vi "Combined Algorithm.vi"() -> ()   [LabVIEW 2020]
uses:
  <vilib>/MakerHub/LINX/Private/Type Defs/Peripherals/SPI/SPI Configuration.ctl
  <vilib>/MakerHub/LINX/Private/Type Defs/Peripherals/SPI/SPI Bit Order.ctl
  <vilib>/MakerHub/LINX/Private/Type Defs/Peripherals/SPI/SPI Mode.ctl
  <vilib>/MakerHub/LINX/Public/Peripherals/SPI/SPI CS Config.ctl
  <vilib>/MakerHub/LINX/Private/Type Defs/Peripherals/SPI/SPI CS Logic Level.ctl
  <vilib>/MakerHub/LINX/Public/Peripherals/Analog/Analog Read 1 Chan.vi
  <vilib>/MakerHub/LINX/Public/Peripherals/Digital/Digital Write 1 Chan.vi
  <vilib>/MakerHub/LINX/Public/Peripherals/SPI/SPI Write Read 1 Frame.vi
  <vilib>/MakerHub/LINX/Public/Peripherals/PWM/PWM Set Duty Cycle 1 Chan.vi
  <vilib>/MakerHub/LINX/Public/Peripherals/Analog/Analog Read N Chans.vi
  <vilib>/MakerHub/LINX/Public/Peripherals/Digital/Digital Write N Chans.vi
  <vilib>/MakerHub/LINX/Public/Peripherals/SPI/SPI Write Read N Frames.vi
  <vilib>/MakerHub/LINX/Private/Local IO/LinxAnalogRead.vi
  <vilib>/MakerHub/LINX/Public/Utilities/Check Channel.vi
  <vilib>/MakerHub/LINX/Private/Local IO/LinxDigitalWrite.vi
  <vilib>/MakerHub/LINX/Private/Local IO/LinxSpiWriteRead.vi
  <vilib>/MakerHub/LINX/Public/Utilities/Open Serial.vi
  <vilib>/MakerHub/LINX/Private/Utilties/Generate Error.vi
  <vilib>/MakerHub/LINX/Public/Peripherals/PWM/PWM Set Duty Cycle N Chans.vi
  <vilib>/MakerHub/LINX/LMH-LINX.lvlib
panel:
  in  "Esp32 SMS Send":u8
  out "LCD Response":u8[](array[numeric])
  in  "IR Sensor Analog Channel 2":u8
  in  "DO Channel -  Exhaust Fan":u8
  in  "DO Channel - Solar Water Motor":u8
  in  "IR sensor Analog Channel (A0)":u8
  out "IR Sensor (Fire detected)":bool
  out "IR Sensor output voltage":dbl
  in  "PWM Channel - Buzzer":u8
  in  "Smoke Threshold":dbl
  out "Smoke sensor output Voltage":dbl
  in  "Smoke sensor Analog Channel(A2)":u8
  out "Temperature":dbl
  in  "stop":bool
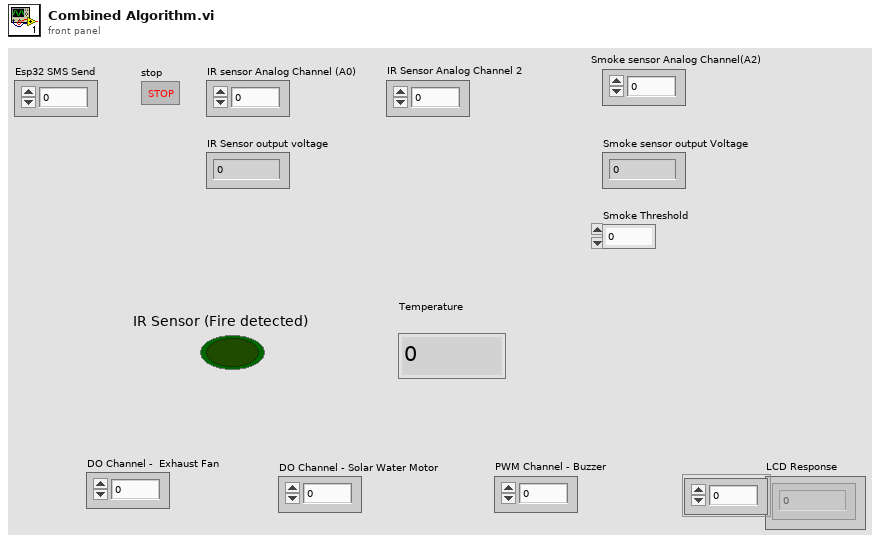
[diagram p1: front panel]
types:
  T1 = typedef "LMH-LINX.lvlib/SPI Configuration.ctl" = cluster{"Clock Frequency":u32, "Bit Order":T2, "SPI Mode":T3}
  T2 = typedef "LMH-LINX.lvlib/SPI Bit Order.ctl" = enum8{"LSb First", "MSb First"}
  T3 = typedef "LMH-LINX.lvlib/SPI Mode.ctl" = enum8{"Mode 0", "Mode 1", "Mode 2", "Mode 3"}
  T4 = typedef "LMH-LINX.lvlib/LINX Ref.ctl" = cluster{"IO":T5, "Interface":T6, "LINX Device Config":T7}
  T5 = typedef "LMH-LINX.lvlib/Platform.ctl" = enum16{"Remote", "Local"}
  T6 = typedef "LMH-LINX.lvlib/Interface.ctl" = enum16{"Serial", "TCP"}
  T7 = typedef "LMH-LINX.lvlib/Device.lvlib/LINX Device Config.ctl" = cluster{"Interface":T6, "COM Port":refnum<visa-resource-name>, "TCP Configuration":T8, "Device Family":u8, "Device ID":u8, "Device Name":string, "TCP Ref":refnum<k5>, "Channels":T9}
  T8 = typedef "LMH-LINX.lvlib/Device.lvlib/TCP Config.ctl" = cluster{"IP Address":string, "Port":u16}
  T9 = typedef "LMH-LINX.lvlib/Channels.ctl" = cluster{"DI":u8[], "DO":u8[], "AI":u8[], "AO":u8[], "PWM":u8[], "QE":u8[], "UART":u8[], "I2C 2":u8[], "SPI":u8[], "CAN":u8[], "Servo":u8[], "AI Ref (V)":dbl, "AI Resolution (Bits)":u8, "AO Ref (V)":dbl, "AO Resolution (Bits)":u8}
  T10 = typedef "LMH-LINX.lvlib/SPI CS Config.ctl" = cluster{"CS Channel":u8, "CS Logic Level":T11}
  T11 = typedef "LMH-LINX.lvlib/SPI CS Logic Level.ctl" = enum8{"Active Low", "Active High"}
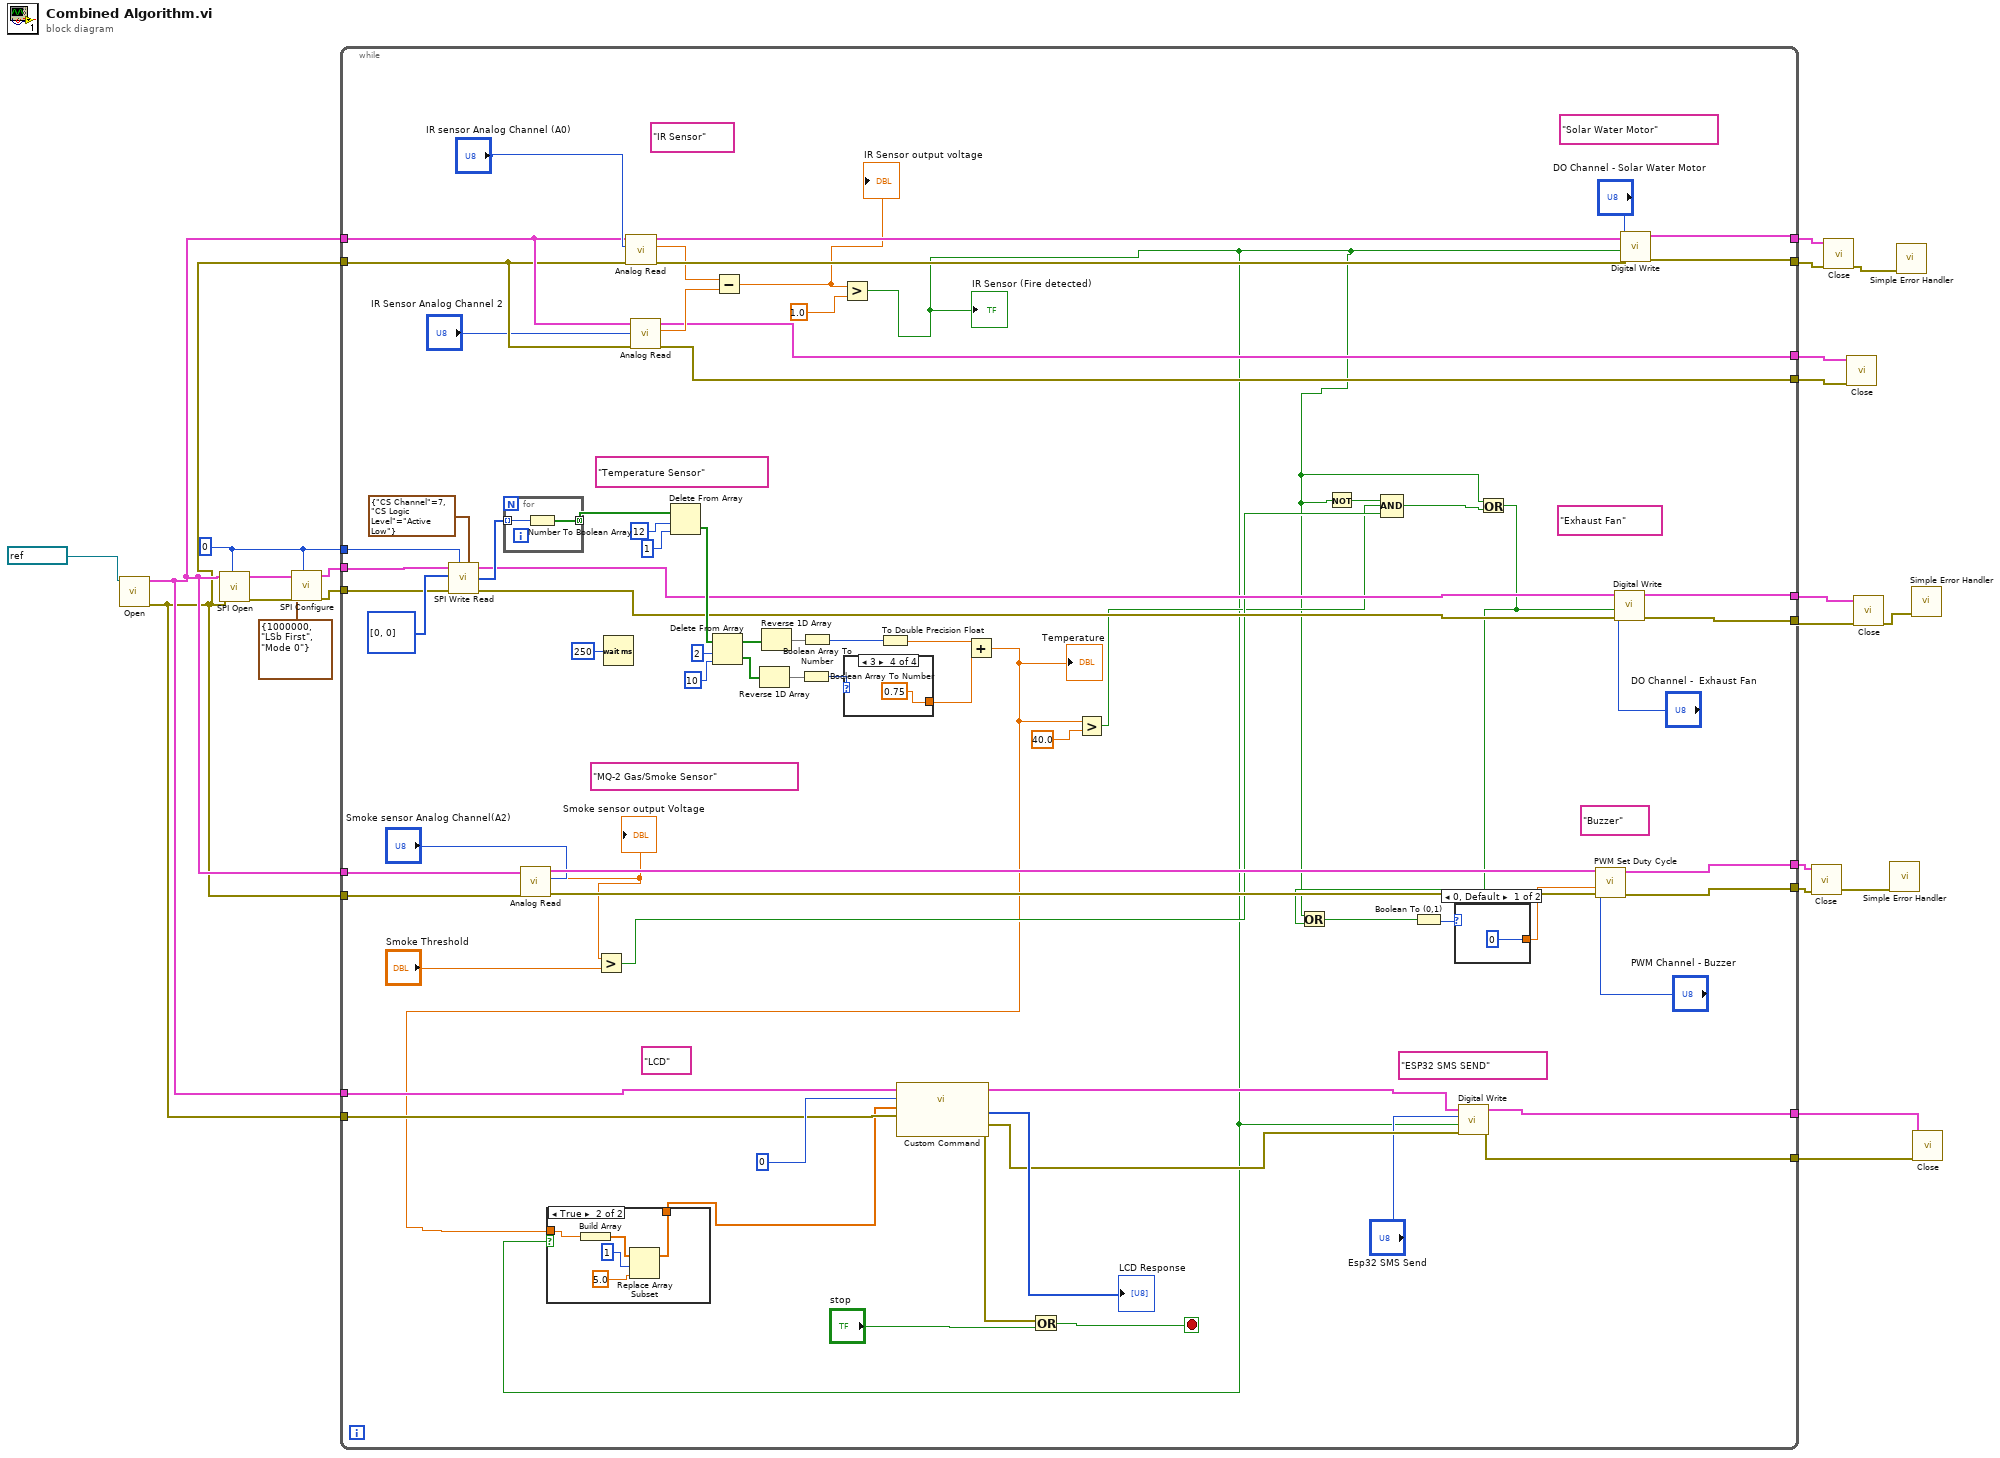
[diagram p0: block diagram]
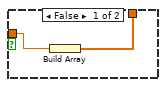
[diagram p2: hidden frame]
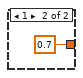
[diagram p3: hidden frame]
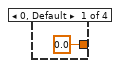
[diagram p4: hidden frame]
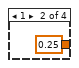
[diagram p5: hidden frame]
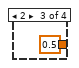
[diagram p6: hidden frame]
diagram:
  w16 = u8 0 ("SPI Channel (0)")
  n1 = call-poly <vilib>:"Open.vi"("Serial Port"=refnum<visa-resource-name> "COM3") -> ("Error Out"=w3:errorcluster, "LINX Resource"=w4:T4)  [unwired: 8 in, 1 out]
  n2 = call <vilib>:"SPI Open.vi"("SPI Channel (0)"=w16, "Error In"=w3, "LINX Resource"=w4) -> ("Error Out"=w21:errorcluster, "LINX Resource"=w20:T4)  [unwired: 7 in]
  n3 = call <vilib>:"SPI Configure.vi"("SPI Channel (0)"=w16, "Error In"=w21, "SPI Configuration"=T1 {"Clock Frequency"=1000000, "Bit Order"=enum."LSb First", "SPI Mode"=enum."Mode 0"}, "LINX Resource"=w20) -> ("Error Out"=w18:errorcluster, "LINX Resource"=w19:T4)  [unwired: 5 in, 1 out]
  n4 = while {
    tunnel: w19 -> [w95]
    tunnel: [w56] -> w10
    tunnel: w18 -> [w78]
    tunnel: [w55] -> w17
    tunnel: w16 -> [w77]
    tunnel: w4 -> [w69]
    tunnel: w3 -> [w68]
    tunnel: [w66] -> w14
    tunnel: [w65] -> w13
    tunnel: w4 -> [w46]
    tunnel: w3 -> [w45]
    tunnel: [w61] -> w12
    tunnel: [w60] -> w11
    tunnel: [w40] -> w6
    tunnel: [w39] -> w5
    tunnel: w4 -> [w34]
    tunnel: w3 -> [w33]
    tunnel: [w27] -> w2
    tunnel: [w29] -> w1
    stop <- w32 stop-if-true
    (unwired) "ESP32 SMS SEND"
    (unwired) "LCD"
    (unwired) "Exhaust Fan"
    (unwired) "Buzzer"
    (unwired) "Solar Water Motor"
    (unwired) "IR Sensor"
    (unwired) "Temperature Sensor"
    (unwired) "MQ-2 Gas/Smoke Sensor"
    n5 = call-poly <vilib>:"SPI Write Read.vi"("CS Configuration"=T10 {"CS Channel"=7, "CS Logic Level"=enum."Active Low"}, "SPI Channel (0)"=w77, "Error In"=w78, "Data"=u16[] [0, 0], "LINX Resource"=w95) -> ("Error Out"=w57:errorcluster, "Read Data"=w93:u8[], "LINX Resource"=w58:T4)  [unwired: 3 in, 1 out]
    n6 = for {
      tunnel: w93 -> [w111] mode=indexing
      tunnel: [w110] -> w76 mode=concatenating
      n7 = Number To Boolean Array(number=w111) -> (Boolean array=w110:bool[])
    }
    n8 = call-poly <vilib>:"Analog Read.vi"("Error In"=w68, "Analog Channel"="Smoke sensor Analog Channel(A2)", "LINX Resource"=w69) -> ("Error Out"=w74:errorcluster, "Voltage"=w72:dbl, "LINX Resource"=w75:T4)  [unwired: 5 in, 1 out]
    "Smoke sensor output Voltage" <- w72
    n9 = Greater?(x=w72, y="Smoke Threshold") -> (0:w49:bool)
    n10 = Wait (ms)(milliseconds to wait=u32 250) -> ()  [unwired: 1 out]
    n11 = call-poly <vilib>:"Analog Read.vi"("Error In"=w45, "Analog Channel"="IR sensor Analog Channel (A0)", "LINX Resource"=w46) -> ("Error Out"=w62:errorcluster, "Voltage"=w43:dbl, "LINX Resource"=w63:T4)  [unwired: 5 in, 1 out]
    n12 = call-poly <vilib>:"Analog Read.vi"("Error In"=w45, "Analog Channel"="IR Sensor Analog Channel 2", "LINX Resource"=w46) -> ("Error Out"=w39:errorcluster, "Voltage"=w42:dbl, "LINX Resource"=w40:T4)  [unwired: 5 in, 1 out]
    n13 = Delete From Array(array=w76, length=12, index=1) -> (deleted portion=w89:bool[])  [unwired: 1 out]
    n14 = Delete From Array(array=w89, length=2, index=10) -> (deleted portion=w85:bool[], array with subset deleted=w86:bool[])
    n15 = Subtract(x=w43, y=w42) -> (x-y=w41:dbl)
    "IR Sensor output voltage" <- w41
    n16 = Reverse 1D Array(array=w85) -> (reversed array=w83:bool[])
    n17 = Reverse 1D Array(array=w86) -> (reversed array=w84:bool[])
    n18 = Boolean Array To Number(Boolean array=w83) -> (number=w82:u32)
    n19 = Boolean Array To Number(Boolean array=w84) -> (number=w79:u32)
    n20 = Greater?(x=w41, y=1.0) -> (0:w23:bool)
    "IR Sensor (Fire detected)" <- w23
    n21 = case shown="3" w82 {
      tunnel: [0.0 0.25 0.5 0.75] -> w81
      frame 0, Default {
      }
      frame 1 {
      }
      frame 2 {
      }
      frame 3 {
      }
    }
    n22 = To Double Precision Float(number=w79) -> (double precision float=w80:dbl)
    n23 = Add(x=w80, y=w81) -> (x+y=w24:dbl)
    "Temperature" <- w24
    n24 = case shown="True" w23 {
      tunnel: w24 -> [w98 w101]
      tunnel: [w97 w99] -> w25
      frame False {
        n25 = Build Array(w98) -> (w97:dbl[])
      }
      frame True {
        n26 = Build Array(w101) -> (w100:dbl[])
        n27 = Replace Array Subset(array=w100, new element=5.0 ("new element/subarray"), index=1) -> (w99:dbl[])
      }
    }
    n28 = call <vilib>:"Custom Command.vi"("Error In"=w33, "Data"=w25, "Custom Command Number"=u16 0, "LINX Resource"=w34) -> ("Error Out"=w28:errorcluster, "Response"=→"LCD Response":u8[], "LINX Resource"=w30:T4)  [unwired: 4 in, 1 out]
    n29 = Or(x=w28, y="stop") -> (x .or. y?=w32:bool)
    n30 = Greater?(x=w24, y=40.0) -> (0:w48:bool)
    n31 = Not(x=w23) -> (.not. x?=w50:bool)
    n32 = Compound Arithmetic op=AND(w50, w48, w49) -> (w38:bool)
    n33 = call-poly <vilib>:"Digital Write.vi"("Error In"=w28, "Output Value"=w23, "DO Channel"="Esp32 SMS Send", "LINX Resource"=w30) -> ("Error Out"=w27:errorcluster, "LINX Resource"=w29:T4)  [unwired: 6 in]
    n34 = Or(x=w23, y=w38) -> (x .or. y?=w37:bool)
    n35 = Or(x=w23, y=w37) -> (x .or. y?=w51:bool)
    n36 = Boolean To (0,1)(Boolean=w51) -> (0, 1=w71:i16)
    n37 = case shown="0, Default" w71 {
      tunnel: [0 0.7] -> w52
      frame 0, Default {
      }
      frame 1 {
      }
    }
    n38 = call-poly <vilib>:"PWM Set Duty Cycle.vi"("Error In"=w74, "Duty Cycle (0-1)"=w52, "PWM Channel"="PWM Channel - Buzzer", "LINX Resource"=w75) -> ("Error Out"=w65:errorcluster, "LINX Resource"=w66:T4)  [unwired: 6 in]
    n39 = call-poly <vilib>:"Digital Write.vi"("Error In"=w57, "Output Value"=w37, "DO Channel"="DO Channel -  Exhaust Fan", "LINX Resource"=w58) -> ("Error Out"=w55:errorcluster, "LINX Resource"=w56:T4)  [unwired: 6 in]
    n40 = call-poly <vilib>:"Digital Write.vi"("Error In"=w62, "Output Value"=w23, "DO Channel"="DO Channel - Solar Water Motor", "LINX Resource"=w63) -> ("Error Out"=w60:errorcluster, "LINX Resource"=w61:T4)  [unwired: 6 in]
  }
  n41 = call <vilib>:"Close.vi"("Error In"=w13, "LINX Resource"=w14) -> ("Error Out"=w9:errorcluster)  [unwired: 9 in]
  n42 = call <vilib>:"Close.vi"("Error In"=w11, "LINX Resource"=w12) -> ("Error Out"=w7:errorcluster)  [unwired: 9 in]
  n43 = call <vilib>:"Close.vi"("Error In"=w5, "LINX Resource"=w6) -> ()  [unwired: 9 in, 1 out]
  n44 = call <vilib>:"Close.vi"("Error In"=w17, "LINX Resource"=w10) -> ("Error Out"=w8:errorcluster)  [unwired: 9 in]
  n45 = call <vilib>:"Simple Error Handler.vi"("error in (no error)"=w9) -> ()  [unwired: 4 in, 5 out]
  n46 = call <vilib>:"Simple Error Handler.vi"("error in (no error)"=w7) -> ()  [unwired: 4 in, 5 out]
  n47 = call <vilib>:"Simple Error Handler.vi"("error in (no error)"=w8) -> ()  [unwired: 4 in, 5 out]
  n48 = call <vilib>:"Close.vi"("Error In"=w2, "LINX Resource"=w1) -> ()  [unwired: 9 in, 1 out]
